vi "MachineGUID.vi"(8 "error in (no error)":errorcluster) -> (0 "error out":errorcluster, 3 "Machine GUID":string)   [LabVIEW 2022 SP3, in "MES_Local.lvlib" / "MES_Local.lvclass"]
uses:
  MES_Local.lvclass
  <vilib>/registry/registry.llb/Registry SAM.ctl
  <vilib>/registry/registry.llb/Registry RtKey.ctl
  <vilib>/registry/registry.llb/Registry View.ctl
  <vilib>/registry/registry.llb/Read Registry Value Simple STR.vi
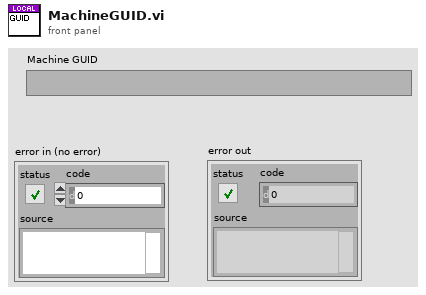
[diagram p1: front panel]
types:
  T1 = typedef "Registry RtKey.ctl" = enum32{"HKEY_CLASSES_ROOT", "HKEY_CURRENT_USER", "HKEY_LOCAL_MACHINE", "HKEY_USERS", "HKEY_PERFORMANCE_DATA", "HKEY_CURRENT_CONFIG", "HKEY_DYN_DATA"}
  T2 = typedef "Registry SAM.ctl" = enum32{"KEY_QUERY_VALUE", "KEY_SET_VALUE", "KEY_CREATE_SUB_KEY", "KEY_ENUMERATE_SUB_KEYS", "KEY_NOTIFY", "KEY_CREATE_LINK", "KEY_READ", "KEY_WRITE", "KEY_ALL_ACCESS", "KEY_READ | KEY_WRITE"}
  T3 = typedef "Registry View.ctl" = u16
  T4 = typedef "Registry refnum.ctl" = refnum<k1>
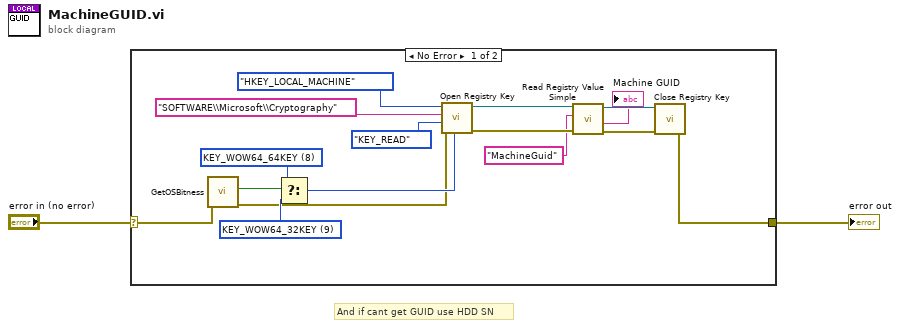
[diagram p0: block diagram]
diagram:
  # "And if cant get GUID use HDD SN"
  n1 = case shown="No Error" "error in (no error)" {
    selector: "error in (no error)" -> [w3 w19]
    tunnel: [w4 w19] -> w2
    frame No Error {
      w7 = T3 9 items=["Default"=0, "KEY_WOW64_64KEY"=8, "KEY_WOW64_32KEY"=9] ("registry view")
      w8 = T3 8 items=["Default"=0, "KEY_WOW64_64KEY"=8, "KEY_WOW64_32KEY"=9] ("registry view")
      n2 = call "GetOSBitness.vi"("error in (no error)"=w3) -> ("error out"=w5:errorcluster, "64-bit system"=w9:bool)  [unwired: 9 in]
      n3 = Select(t=w8, s=w9, f=w7) -> (s? t:f=w6:T3)
      n4 = call <vilib>:"Open Registry Key.vi"("registry view"=w6, "error in (no error)"=w5, "security access mask (KEY_READ | KEY_WRITE)"=Registry_SAM."KEY_READ", "subkey"="SOFTWARE\\Microsoft\\Cryptography", "root key (HKEY_LOCAL_MACHINE)"=Registry_RtKey."HKEY_LOCAL_MACHINE") -> ("error out"=w18:errorcluster, "refnum out"=w11:T4)  [unwired: 5 in]
      n5 = call-poly <vilib>:"Read Registry Value Simple.vi"("error in (no error)"=w18, "value"="MachineGuid", "refnum"=w11) -> ("error out"=w17:errorcluster, "String/Binary data"=→"Machine GUID":string, "refnum out"=w16:T4)  [unwired: 3 in, 1 out]
      n6 = call <vilib>:"Close Registry Key.vi"("error in (no error)"=w17, "refnum"=w16) -> ("error out"=w4:errorcluster)  [unwired: 5 in]
    }
    frame Error {
    }
  }
  "error out" <- w2
